vi "newgauge.vi"() -> ()   [LabVIEW 2018]
panel:
  out "error out":errorcluster
  out "read buffer":string
  out "return count":u32
  in  "VISA resource name":refnum<visa-resource-name>
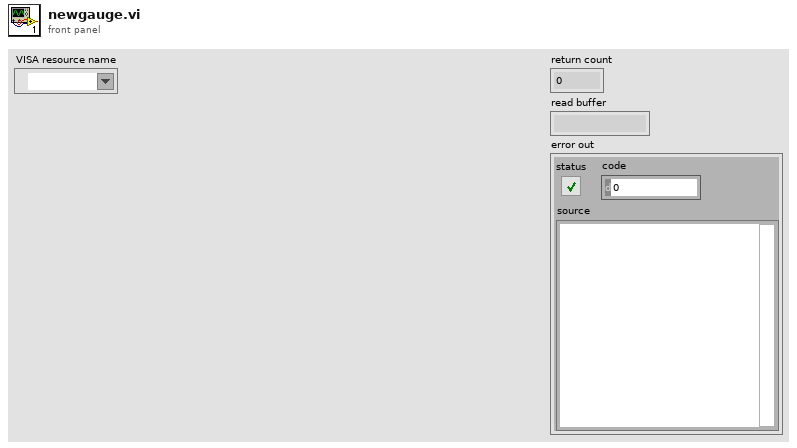
[diagram p1: front panel]
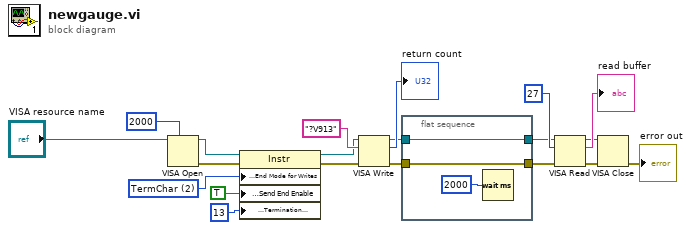
[diagram p0: block diagram]
diagram:
  w7 = u16 2 items=["None", "Last Bit", "TermChar", "Break"] ("Serial Settings:End Mode for Writes")
  n1 = VISA Open(timeout (0)=u32 2000 ("VISA Open timeout (0)"), VISA resource name="VISA resource name") -> (VISA resource name=w4:refnum<visa-resource-name>, error out=w3:errorcluster)  [unwired: 3 in]
  n2 = property class="Instr"(reference=w4, error in=w3, "Serial Settings:End Mode for Writes"=w7, "Message Based Settings:Send End Enable"=TRUE, "Message Based Settings:Termination Character"=u8 13) -> (reference out=w1:refnum<visa-resource-name>, error out=w2:errorcluster)
  n3 = VISA Write(VISA resource name=w1, write buffer="?V913", error in (no error)=w2) -> (VISA resource name out=w15:refnum<visa-resource-name>, return count=→"return count":u32, error out=w13:errorcluster)
  n4 = flat-sequence {
    tunnel: w15 -> [w23]
    tunnel: [w23] -> w9
    tunnel: w13 -> [w21]
    tunnel: [w21] -> w12
    frame #0 {
      n5 = Wait (ms)(milliseconds to wait=u32 2000) -> ()  [unwired: 1 out]
    }
  }
  n6 = VISA Read(VISA resource name=w9, byte count=u32 27, error in (no error)=w12) -> (VISA resource name out=w14:refnum<visa-resource-name>, read buffer=→"read buffer":string, error out=w11:errorcluster)  [unwired: 1 out]
  n7 = VISA Close(VISA resource name=w14, error in (no error)=w11) -> (error out=→"error out":errorcluster)
